vi "transform_to_rvec_pose.vi"(10 "Transform":T1) -> (2 "Rotation vector pose":dbl[][](array[numeric]))   [LabVIEW 2024]
uses:
  <vilib>/Analysis/Matrix/Datatypes/RealMatrix.ctl
  <vilib>/Analysis/NI_AALPro.lvlib
  <vilib>/Analysis/7linalg.llb/Create Special Real Matrix.vi
  <vilib>/Analysis/_algsub.llb/Real Matrix Trace.vi
  <vilib>/Analysis/Matrix/NI_Matrix.lvlib
  <vilib>/Analysis/Matrix/Numeric/Subtract/Subtract - RM,RM.vi
panel:
  # "Convert 4x4 linear homogenous pose representation into X Y Z Rx Ry Rz where the rotation part is the rotation axis scaled by the rotation magnitude (in radians). This is not Euler angles."
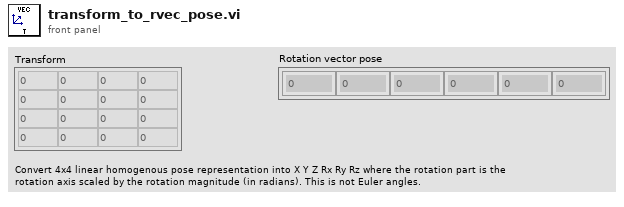
[diagram p1: front panel]
types:
  T1 = typedef "NI_Matrix.lvlib/RealMatrix.ctl" = dbl[][]
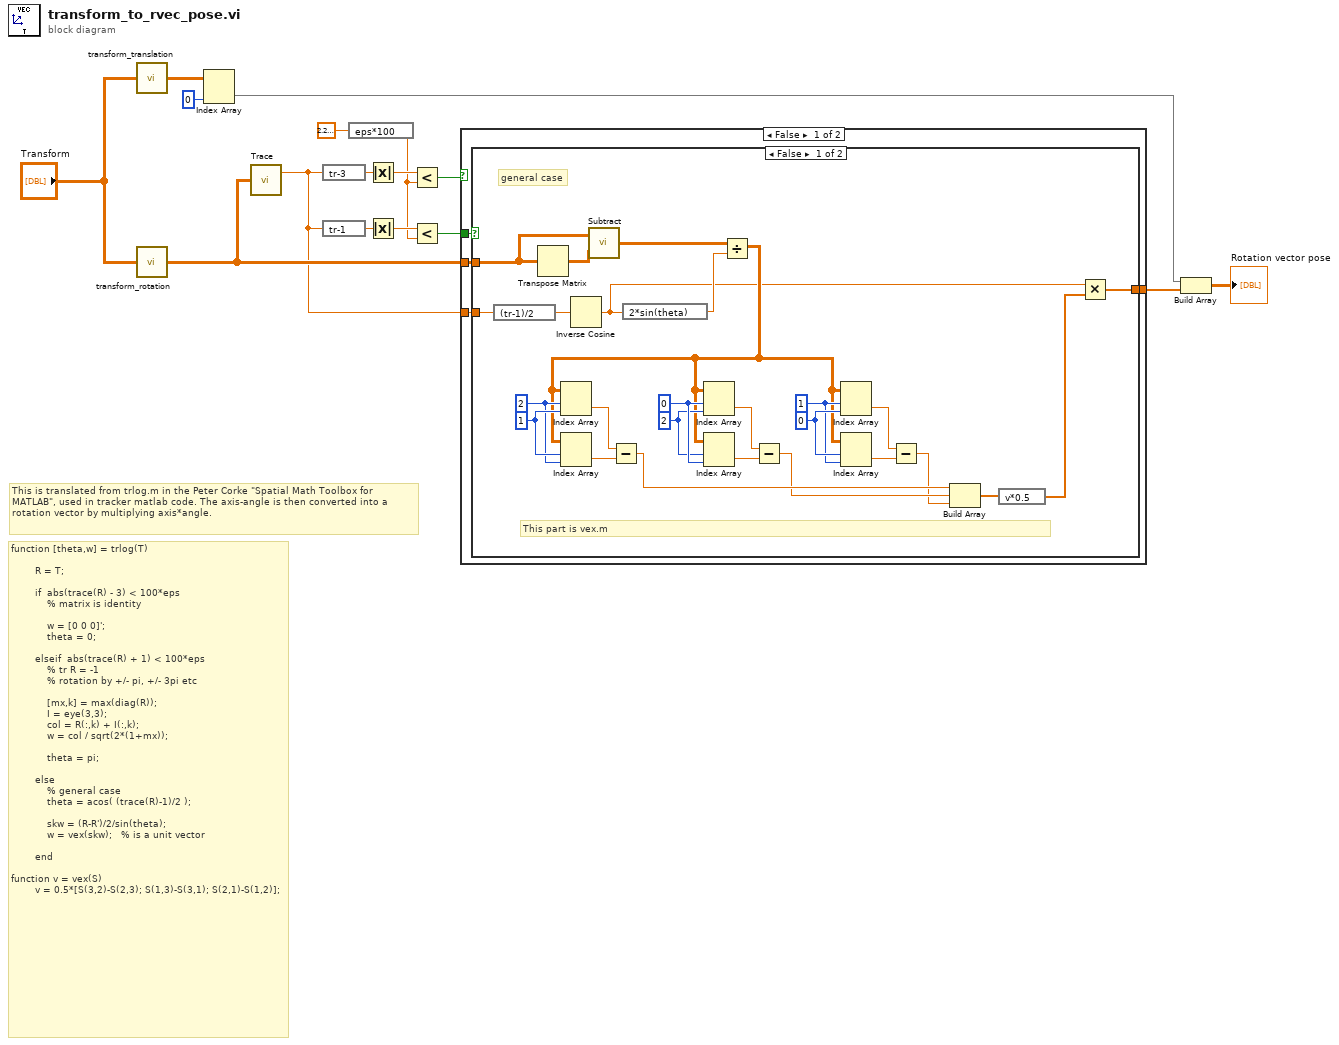
[diagram p0: block diagram]
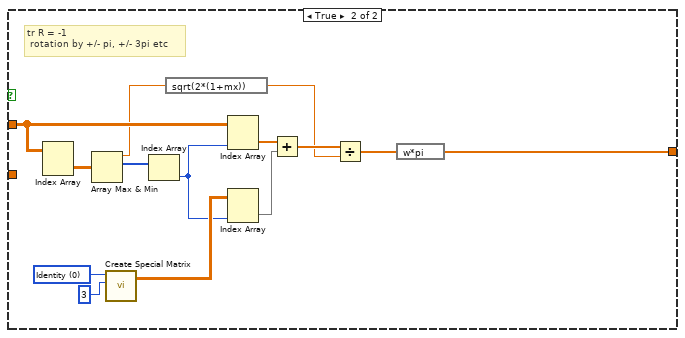
[diagram p2: hidden frame]
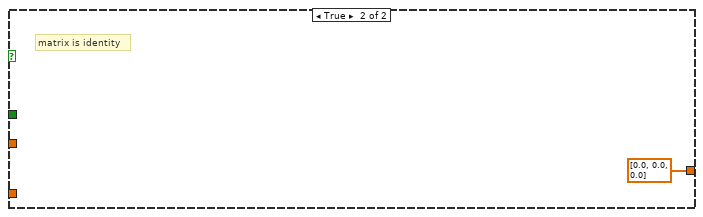
[diagram p3: hidden frame]
diagram:
  # "function [theta,w] = trlog(T)\n        \n        R = T;\n        \n        if  abs(trace(R) - 3) < 100*eps\n            % matrix is identity\n            \n            w = [0 0 0]';\n            theta = 0;\n            \n        elseif  abs(trace(R) + 1) < 100*eps\n            % tr R = -1\n            % rotation by +/- pi, +/- 3pi etc\n            \n            [mx,k] = max(diag(R));\n            I = eye(3,3);\n            col = R(:,k) + I(:,k);\n            w = col / sqrt(2*(1+mx));\n            \n            theta = pi;\n     \n        else\n            % general case\n            theta = acos( (trace(R)-1)/2 );\n            \n            skw = (R-R')/2/sin(theta);\n            w = vex(skw);   % is a unit vector\n            \n        end\n\nfunction v = vex(S)\n        v = 0.5*[S(3,2)-S(2,3); S(1,3)-S(3,1); S(2,1)-S(1,2)];"
  # "This is translated from trlog.m in the Peter Corke \"Spatial Math Toolbox for MATLAB\", used in tracker matlab code. The axis-angle is then converted into a rotation vector by multiplying axis*angle."
  n1 = call "transform_translation.vi"("Transform"="Transform") -> ("Translation"=w3:T1)  [unwired: 4 in]
  n2 = call "transform_rotation.vi"("Transform"="Transform") -> ("Rotation"=w6:T1)  [unwired: 4 in]
  n3 = Index Array(array=w3, index (col)=0 ("disabled index (col)")) -> (element=w2:dbl[])  [unwired: 1 in]
  n4 = call-poly <vilib>:"Trace.vi"("Input Matrix"=w6) -> ("trace"=w5:dbl)  [unwired: 1 out]
  n5 = expression code="tr-3"(w5) -> (w15:dbl)
  n6 = expression code="tr-1"(w5) -> (w12:dbl)
  n7 = expression code="eps*100"(2.220446049250313e-16) -> (w11:dbl)
  n8 = Absolute Value(x=w15) -> (abs(x)=w14:dbl)
  n9 = Absolute Value(x=w12) -> (abs(x)=w13:dbl)
  n10 = Less?(x=w14, y=w11) -> (x < y?=w10:bool)
  n11 = Less?(x=w13, y=w11) -> (x < y?=w7:bool)
  n12 = case shown="False" w10 {
    tunnel: [w18 dbl[] [0.0, 0.0, 0.0]] -> w8
    tunnel: w7 -> [w20 _]
    tunnel: w6 -> [w19 _]
    tunnel: w5 -> [w17 _]
    frame False {
      n13 = case shown="False" w20 {
        tunnel: w19 -> [w43 w57]
        tunnel: [w22 w47] -> w18
        tunnel: w17 -> [w46 _]
        frame False {
          w32 = 0 ("disabled index (col)")
          w31 = 1 ("index (row)")
          w33 = 2 ("disabled index (col)")
          w34 = 0 ("index (row)")
          w40 = 1 ("disabled index (col)")
          w39 = 2 ("index (row)")
          # "This part is vex.m"
          # "general case"
          n14 = expression code="(tr-1)/2"(w46) -> (w45:dbl)
          n15 = Transpose Matrix(1:w43) -> (0:w44:T1)
          n16 = Inverse Cosine(1:w45) -> (0:w21:dbl)
          n17 = call-poly <vilib>:"Subtract.vi"("Real Matrix B"=w44, "Real Matrix A"=w43) -> ("A - B"=w42:T1)
          n18 = expression code="2*sin(theta)"(w21) -> (w41:dbl)
          n19 = Divide(x=w42, y=w41) -> (x/y=w28:T1)
          n20 = Index Array(array=w28, index (row)=w39, index (col)=w40) -> (element=w38:dbl)
          n21 = Index Array(array=w28, index (row)=w40, index (col)=w39) -> (element=w37:dbl)
          n22 = Subtract(x=w38, y=w37) -> (x-y=w27:dbl)
          n23 = Index Array(array=w28, index (row)=w34, index (col)=w33) -> (element=w35:dbl)
          n24 = Index Array(array=w28, index (row)=w33, index (col)=w34) -> (element=w36:dbl)
          n25 = Subtract(x=w35, y=w36) -> (x-y=w26:dbl)
          n26 = Index Array(array=w28, index (row)=w31, index (col)=w32) -> (element=w30:dbl)
          n27 = Index Array(array=w28, index (row)=w32, index (col)=w31) -> (element=w29:dbl)
          n28 = Subtract(x=w30, y=w29) -> (x-y=w25:dbl)
          n29 = Build Array(w27, w26, w25) -> (w24:dbl[])
          n30 = expression code="v*0.5"(w24) -> (w23:dbl[])
          n31 = Multiply(x=w21, y=w23) -> (x*y=w22:dbl[])
        }
        frame True {
          w59 = 0 items=["Identity", "Diagonal", "Toeplitz", "Vandermonde", "Companion", "Hankel", "Hadamard", "Wilkinson", "Hilbert", "Inverse Hilbert", "Rosser", "Pascal"] ("matrix type")
          # "tr R = -1\n rotation by +/- pi, +/- 3pi etc"
          n32 = Index Array(array=w57) -> (element=w60:T1)  [unwired: 2 in]
          n33 = Array Max & Min(array=w60) -> (max value=w50:dbl, max index (indices)=w56:i32[])  [unwired: 2 out]
          n34 = call-poly <vilib>:"Create Special Matrix.vi"("matrix type"=w59, "matrix size"=3) -> ("Special Matrix"=w55:T1)  [unwired: 3 in, 1 out]
          n35 = Index Array(array=w56) -> (element=w54:i32)  [unwired: 1 in]
          n36 = expression code="sqrt(2*(1+mx))"(w50) -> (w49:dbl)
          n37 = Index Array(array=w57, index (col)=w54) -> (element=w53:dbl[])  [unwired: 1 in]
          n38 = Index Array(array=w55, index (col)=w54) -> (element=w52:dbl[])  [unwired: 1 in]
          n39 = Add(x=w53, y=w52) -> (x+y=w51:dbl[])
          n40 = Divide(x=w51, y=w49) -> (x/y=w48:dbl[])
          n41 = expression code="w*pi"(w48) -> (w47:dbl[])
        }
      }
    }
    frame True {
      # "matrix is identity"
    }
  }
  n42 = Build Array(w2, w8) -> (→"Rotation vector pose":dbl[][])
